vi "performaction.vi"(11 "command line arguments":T1) -> (0 "error out":errorcluster)   [LabVIEW 2019]
uses:
  executables/arguments.ctl
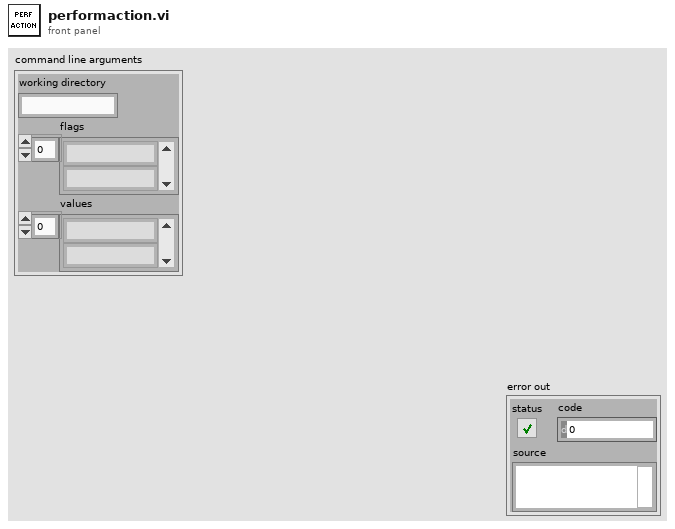
[diagram p1: front panel]
types:
  T1 = typedef "arguments.ctl" = cluster{"working directory":string, "flags":string[], "values":string[]}
  T2 = cluster{"working directory":string, "paths":string[], "args":string[]}
  T3 = cluster{"-noattr":bool, "-nofp":bool, "-nofppos":bool, "-nobd":bool, "-nobdcosm":bool, "-nobdpos":bool}
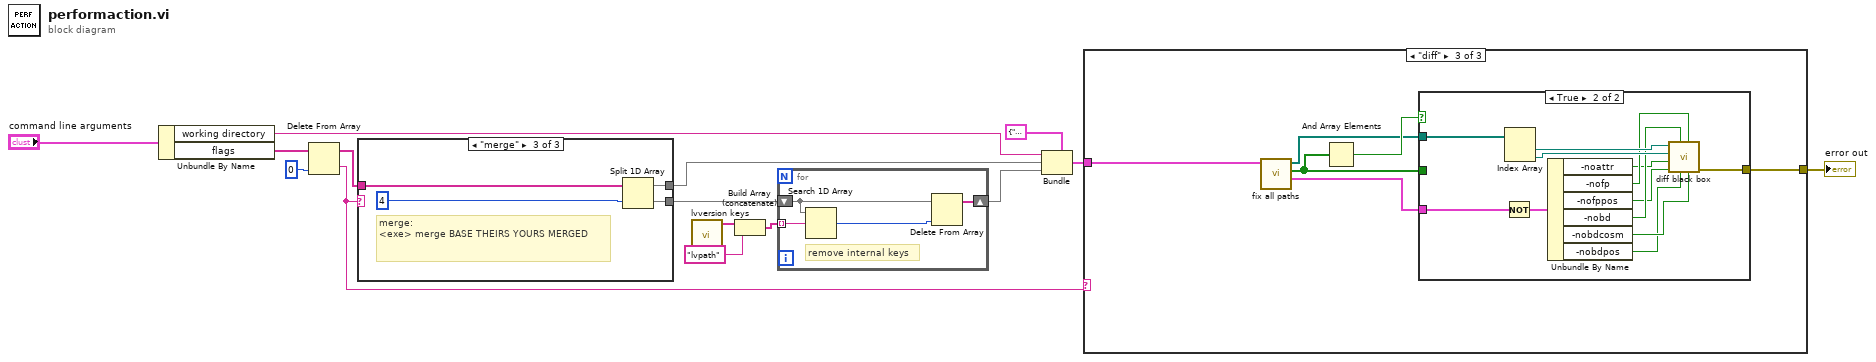
[diagram p0: block diagram]
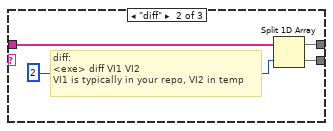
[diagram p3: hidden frame]
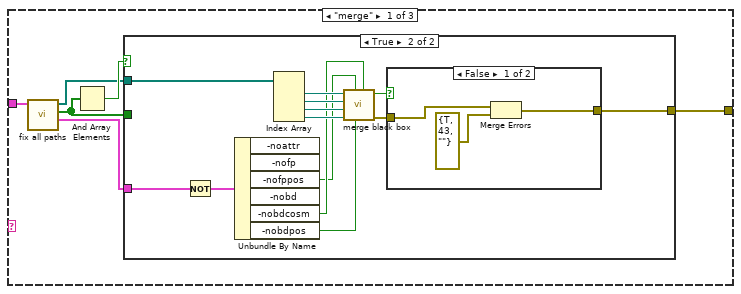
[diagram p4: hidden frame]
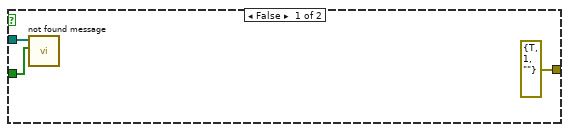
[diagram p5: hidden frame]
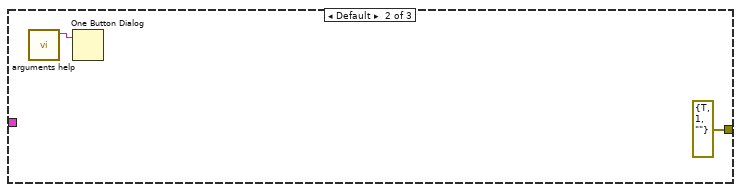
[diagram p7: hidden frame]
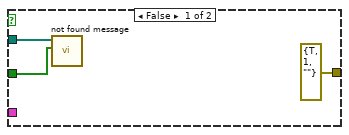
[diagram p8: hidden frame]
diagram:
  n1 = Unbundle By Name("command line arguments") -> ("working directory"=w8:string, "flags"=w12:string[])
  n2 = Delete From Array(array=w12, index=0) -> (deleted portion=w10:string, array with subset deleted=w9:string[])  [unwired: 1 in]
  n3 = case shown="\"merge\"" w10 {
    tunnel: w9 -> [w16 w20 w24]
    tunnel: [_ w18 w22] -> w7
    tunnel: [w16 w17 w21] -> w5
    frame Default {
    }
    frame "diff" {
      # "diff:\n<exe> diff VI1 VI2\nVI1 is typically in your repo, VI2 in temp"
      n4 = Split 1D Array(array=w20, index=2 ("length")) -> (first subarray=w18:string[], second subarray=w17:string[])
    }
    frame "merge" {
      # "merge:\n<exe> merge BASE THEIRS YOURS MERGED"
      n5 = Split 1D Array(array=w24, index=4 ("length")) -> (first subarray=w22:string[], second subarray=w21:string[])
    }
  }
  n6 = call "lvversion keys.vi"() -> ("lv version keys"=w13:string[])  [unwired: 11 in]
  n7 = Build Array (concatenate)(w13, "lvpath" ("String")) -> (w2:string[])
  n8 = for {
    shift-right: [w26] -> w4
    shift-left: w5 -> [w27]
    tunnel: w2 -> [w28] mode=indexing
    # "remove internal keys"
    n9 = Search 1D Array(1D array=w27, element=w28) -> (index of element=w25:i32)  [unwired: 1 in]
    n10 = Delete From Array(array=w27, index=w25) -> (array with subset deleted=w26:string[])  [unwired: 1 in, 1 out]
  }
  n11 = Bundle(cluster=T2 {"working directory"="", "paths"=[], "args"=[]} ("output cluster"), "working directory"=w8, "paths"=w7, "args"=w4) -> (w3:T2)
  n12 = case shown="\"diff\"" w10 {
    tunnel: [w31 errorcluster {"status"=TRUE, "code"=1, "source"=""} ("error out") w59] -> w15
    tunnel: w3 -> [w30 _ w58]
    frame "merge" {
      n13 = call "fix all paths.vi"("paths"=w30) -> ("settings"=w29:T3, "found"=w32:bool[], "paths out"=w33:path[])  [unwired: 8 in]
      n14 = And Array Elements(Boolean array=w32) -> (logical AND=w34:bool)
      n15 = case shown="True" w34 {
        tunnel: w33 -> [w37 w50]
        tunnel: w32 -> [w36 _]
        tunnel: [errorcluster {"status"=TRUE, "code"=1, "source"=""} ("error out") w44] -> w31
        tunnel: w29 -> [_ w42]
        frame False {
          n16 = call "not found message.vi"("found"=w36, "paths in"=w37) -> ()  [unwired: 10 in]
        }
        frame True {
          n17 = Not(x=w42) -> (.not. x?=w38:T3)
          n18 = Unbundle By Name(w38) -> ("-nofppos"=w39:bool, "-nobdcosm"=w40:bool, "-nobdpos"=w41:bool)  [unwired: 3 out]
          n19 = Index Array(array=w50) -> (element #1=w48:path, element #2=w47:path, element #3=w49:path, element #4=w46:path)  [unwired: 4 in]
          n20 = call "merge black box.vi"("BD Cosmetic?"=w40, "BD Pos/Size?"=w41, "FP Pos/Size?"=w39, "merge"=w46, "yours"=w49, "their"=w47, "base"=w48) -> ("error out"=w43:errorcluster, "Saved?"=w45:bool)  [unwired: 3 in]
          n21 = case shown="False" w45 {
            tunnel: [w52 w54] -> w44
            tunnel: w43 -> [w53 w54]
            frame False {
              n22 = Merge Errors(w53, errorcluster {"status"=TRUE, "code"=43, "source"=""} ("error in")) -> (w52:errorcluster)
            }
            frame True {
            }
          }
        }
      }
    }
    frame Default {
      n23 = call "arguments help.vi"() -> ("args help"=w55:string)  [unwired: 11 in]
      n24 = One Button Dialog(message=w55) -> ()  [unwired: 1 in, 1 out]
    }
    frame "diff" {
      n25 = call "fix all paths.vi"("paths"=w58) -> ("settings"=w57:T3, "found"=w60:bool[], "paths out"=w61:path[])  [unwired: 8 in]
      n26 = And Array Elements(Boolean array=w60) -> (logical AND=w62:bool)
      n27 = case shown="True" w62 {
        tunnel: w61 -> [w65 w77]
        tunnel: w60 -> [w64 _]
        tunnel: [errorcluster {"status"=TRUE, "code"=1, "source"=""} ("error out") w74] -> w59
        tunnel: w57 -> [_ w73]
        frame False {
          n28 = call "not found message.vi"("found"=w64, "paths in"=w65) -> ()  [unwired: 10 in]
        }
        frame True {
          n29 = Not(x=w73) -> (.not. x?=w66:T3)
          n30 = Index Array(array=w77) -> (element #1=w76:path, element #2=w75:path)  [unwired: 2 in]
          n31 = Unbundle By Name(w66) -> ("-noattr"=w68:bool, "-nofp"=w70:bool, "-nofppos"=w67:bool, "-nobd"=w69:bool, "-nobdcosm"=w72:bool, "-nobdpos"=w71:bool)
          n32 = call "diff black box.vi"("BD Cosmetic?"=w72, "FP?"=w70, "BD Pos/Size?"=w71, "BD?"=w69, "FP Pos/Size?"=w67, "VI Attributes?"=w68, "VI2 Absolute"=w75, "VI1 Absolute"=w76) -> ("error out"=w74:errorcluster)  [unwired: 3 in]
        }
      }
    }
  }
  "error out" <- w15
